vi "Display Console.vi"(8 "error in (no error)":errorcluster) -> (0 "error out":errorcluster)   [LabVIEW 2017]
uses:
  Type Definitions/Display Data.ctl
  Type Definitions/DB Record.ctl
  Type Definitions/Display Console States.ctl
  Type Definitions/Queue FG Options.ctl
panel:
  out "Card Read":bool
  out "Message Screen":string
  out "Current Transaction":string
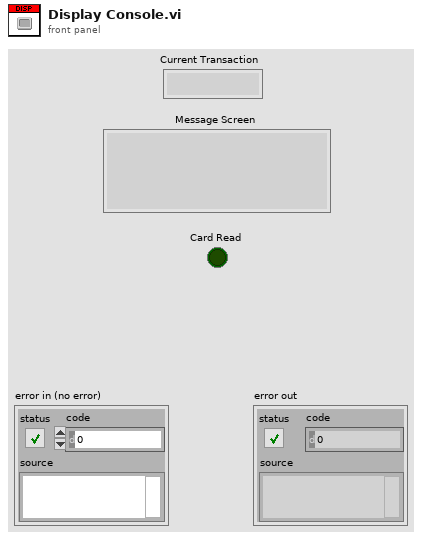
[diagram p1: front panel]
types:
  T1 = typedef "Display Data.ctl" = cluster{"Message Text":string, "DB Record":T2, "Card Read":bool, "Display Console States":T3}
  T2 = typedef "DB Record.ctl" = cluster{"Account":i32, "First Name":string, "Last Name":string, "Balance":fxp<+/-,64,35>}
  T3 = typedef "Display Console States.ctl" = enum16{"Timeout", "Initial", "Login", "Invalid Login", "Idle", "Balance Inquiry", "Deposit", "Withdrawal", "Fast Cash", "Withdrawal Failed", "Withdrawal Complete", "Terminate", "Shutdown"}
  T4 = typedef "Queue FG Options.ctl" = enum16{"Set", "Get", "Read", "Write", "Destroy"}
  T5 = typedef "Display Console Message.ctl" = cluster{"Message Info":T3, "Message Data":variant}
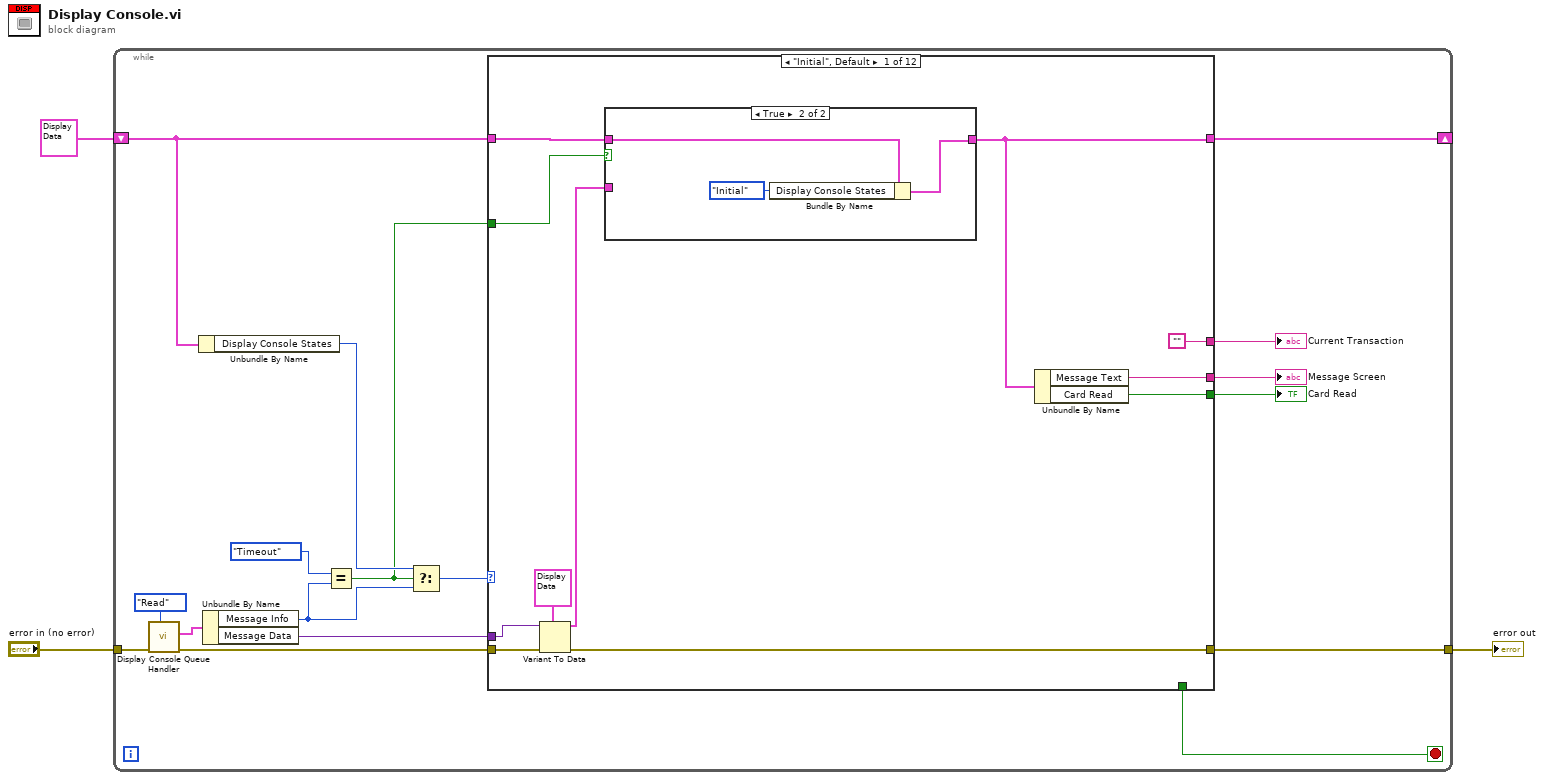
[diagram p0: block diagram]
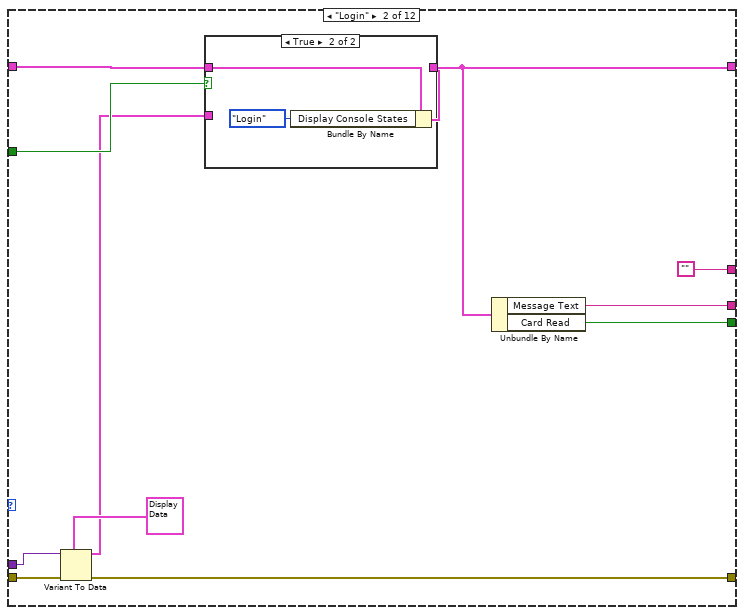
[diagram p3: hidden frame]
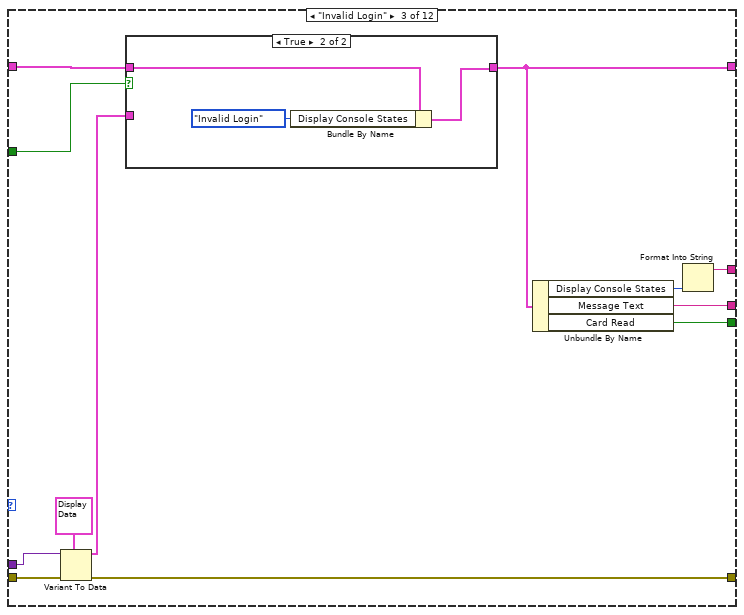
[diagram p5: hidden frame]
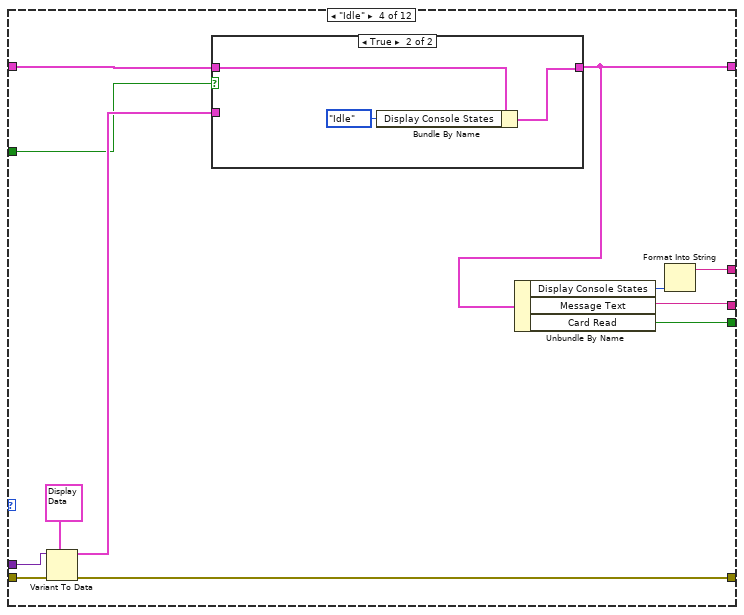
[diagram p7: hidden frame]
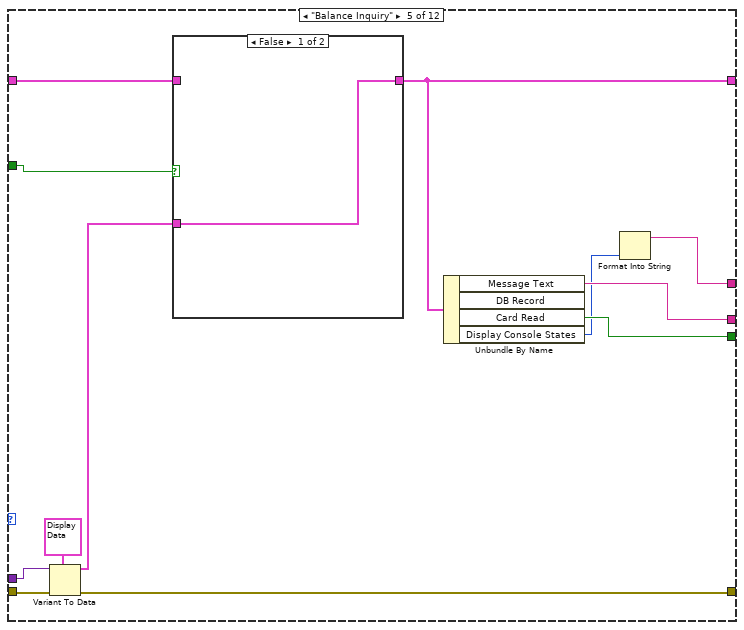
[diagram p9: hidden frame]
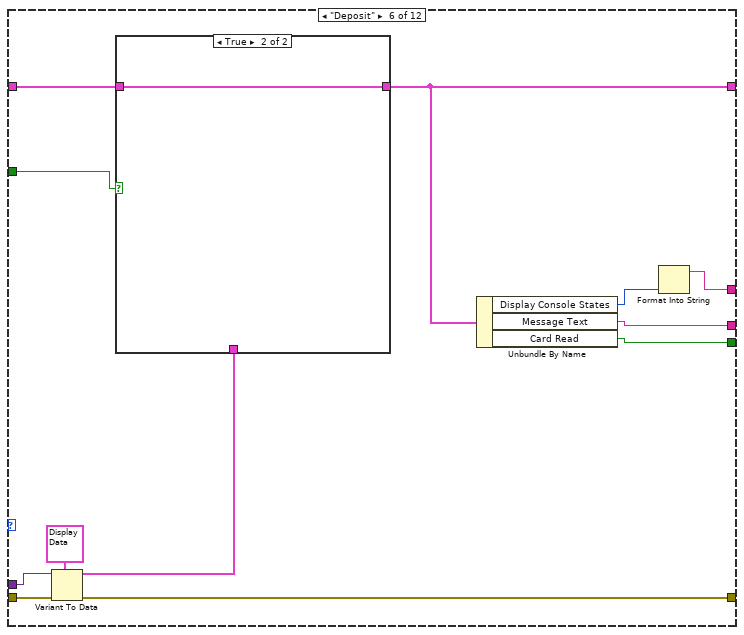
[diagram p11: hidden frame]
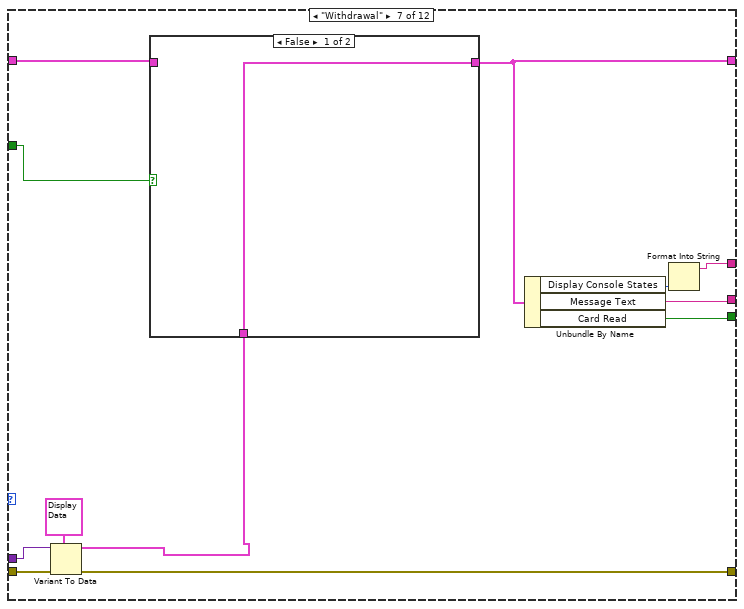
[diagram p13: hidden frame]
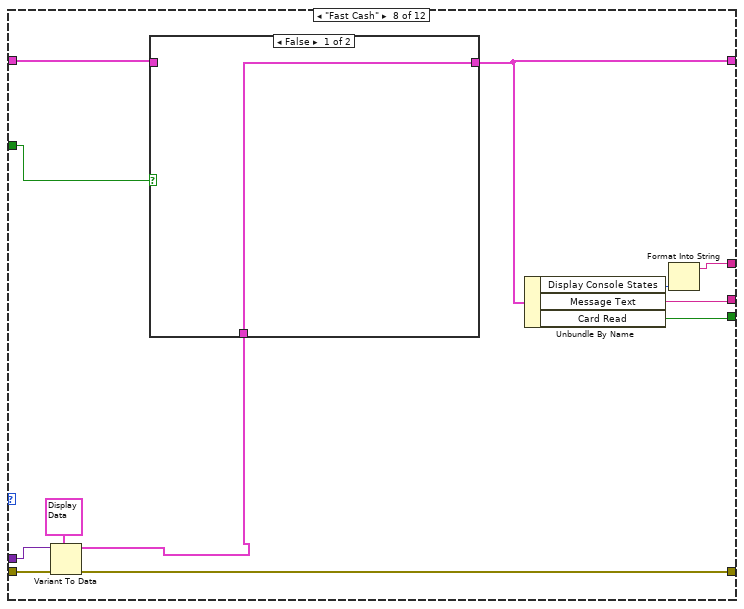
[diagram p15: hidden frame]
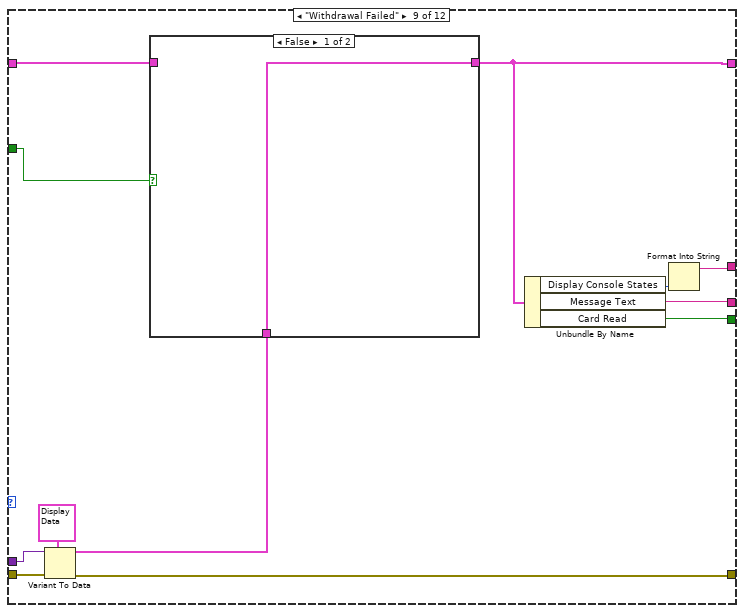
[diagram p17: hidden frame]
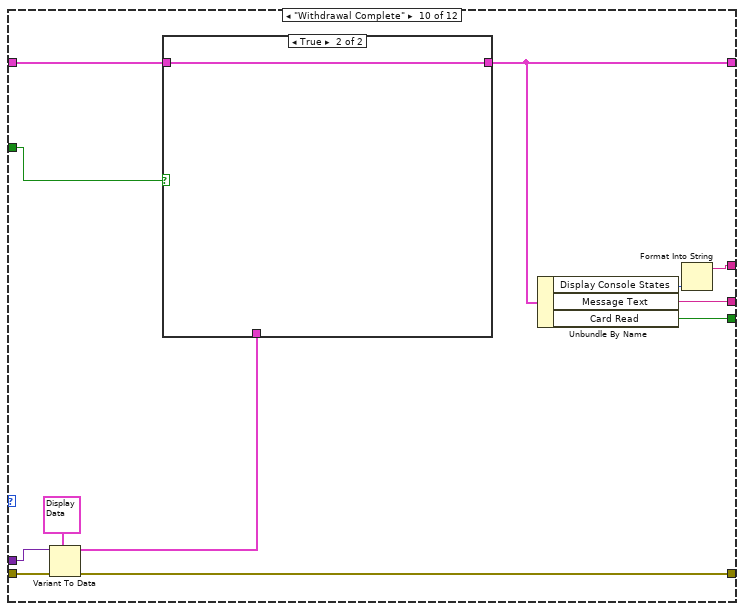
[diagram p19: hidden frame]
diagram:
  n1 = while {
    tunnel: "error in (no error)" -> [w19]
    tunnel: [w15] -> w2
    shift-right: [w10] -> _
    shift-left: T1 {"Message Text"="", "DB Record"={"Account"=0, "First Name"="", "Last Name"="", "Balance"=0.0}, "Card Read"=FALSE, "Display Console States"=enum."Timeout"} ("Display Data") -> [w5]
    stop <- w14 stop-if-true
    n2 = call "Display Console Queue Handler.vi"("Action"=Queue_FG_Options."Read", "error in (no error)"=w19) -> ("error out"=w16:errorcluster, "Message out"=w18:T5)  [unwired: 7 in, 1 out]
    n3 = Unbundle By Name(w5) -> ("Display Console States"=w6:T3)
    n4 = Unbundle By Name(w18) -> ("Message Info"=w8:T3, "Message Data"=w17:variant)
    n5 = Equal?(x=Display_Console_States."Timeout" ("Display Console States"), y=w8) -> (x = y?=w4:bool)
    n6 = Select(t=w6, s=w4, f=w8) -> (s? t:f=w7:T3)
    n7 = case shown="\"Initial\", Default" w7 {
      selector: w7 -> [_ _ _ _ _ _ _ _ _ _ _ w186]
      tunnel: w17 -> [w31 w46 w62 w75 w91 w105 w119 w133 w147 w161 w175 w185]
      tunnel: w16 -> [w30 w45 w61 w77 w93 w107 w121 w135 w149 w163 w177 w188]
      tunnel: [w29 w44 w60 w76 w92 w106 w120 w134 w148 w162 w176 w187] -> w15
      tunnel: [_ _ _ _ _ _ _ _ _ _ _ TRUE] -> w14
      tunnel: [w26 w41 w57 w69 w85 w100 w113 w127 w141 w154 w168 w183] -> w13
      tunnel: ["" "" w51 w70 w83 w97 w114 w128 w142 w155 w169 w182] -> w12
      tunnel: [w27 w42 w58 w68 w86 w99 w112 w126 w140 w153 w167 w184] -> w11
      tunnel: w5 -> [w24 w39 w55 w74 w90 w104 w116 w130 w145 w160 w174 w181]
      tunnel: [w22 w37 w53 w71 w87 w101 w115 w129 w143 w157 w171 w181] -> w10
      tunnel: w4 -> [w25 w40 w56 w67 w89 w102 w111 w125 w144 w158 w172 _]
      frame "Initial", Default {
        n8 = Variant To Data(error in=w30, type=T1 {"Message Text"="", "DB Record"={"Account"=0, "First Name"="", "Last Name"="", "Balance"=0.0}, "Card Read"=FALSE, "Display Console States"=enum."Timeout"} ("Display Data"), Variant=w31) -> (data=w23:T1, error out=w29:errorcluster)
        n9 = case shown="True" w25 {
          tunnel: w24 -> [_ w35]
          tunnel: [w32 w33] -> w22
          tunnel: w23 -> [w32 _]
          frame False {
          }
          frame True {
            n10 = Bundle By Name(cluster=w35, "Display Console States"=Display_Console_States."Initial") -> (w33:T1)
          }
        }
        n11 = Unbundle By Name(w22) -> ("Message Text"=w26:string, "Card Read"=w27:bool)
      }
      frame "Login" {
        n12 = Variant To Data(error in=w45, type=T1 {"Message Text"="", "DB Record"={"Account"=0, "First Name"="", "Last Name"="", "Balance"=0.0}, "Card Read"=FALSE, "Display Console States"=enum."Timeout"} ("Display Data"), Variant=w46) -> (data=w38:T1, error out=w44:errorcluster)
        n13 = case shown="True" w40 {
          tunnel: w39 -> [_ w50]
          tunnel: [w47 w48] -> w37
          tunnel: w38 -> [w47 _]
          frame False {
          }
          frame True {
            n14 = Bundle By Name(cluster=w50, "Display Console States"=Display_Console_States."Login") -> (w48:T1)
          }
        }
        n15 = Unbundle By Name(w37) -> ("Message Text"=w41:string, "Card Read"=w42:bool)
      }
      frame "Invalid Login" {
        n16 = Variant To Data(error in=w61, type=T1 {"Message Text"="", "DB Record"={"Account"=0, "First Name"="", "Last Name"="", "Balance"=0.0}, "Card Read"=FALSE, "Display Console States"=enum."Timeout"} ("Display Data"), Variant=w62) -> (data=w54:T1, error out=w60:errorcluster)
        n17 = case shown="True" w56 {
          tunnel: w55 -> [_ w66]
          tunnel: [w63 w64] -> w53
          tunnel: w54 -> [w63 _]
          frame False {
          }
          frame True {
            n18 = Bundle By Name(cluster=w66, "Display Console States"=Display_Console_States."Invalid Login") -> (w64:T1)
          }
        }
        n19 = Unbundle By Name(w53) -> ("Display Console States"=w52:T3, "Message Text"=w57:string, "Card Read"=w58:bool)
        n20 = Format Into String(w52) -> (resulting string=w51:string)  [unwired: 3 in, 1 out]
      }
      frame "Idle" {
        n21 = Variant To Data(error in=w77, type=T1 {"Message Text"="", "DB Record"={"Account"=0, "First Name"="", "Last Name"="", "Balance"=0.0}, "Card Read"=FALSE, "Display Console States"=enum."Timeout"} ("Display Data"), Variant=w75) -> (data=w73:T1, error out=w76:errorcluster)
        n22 = case shown="True" w67 {
          tunnel: w74 -> [_ w82]
          tunnel: [w79 w80] -> w71
          tunnel: w73 -> [w79 _]
          frame False {
          }
          frame True {
            n23 = Bundle By Name(cluster=w82, "Display Console States"=Display_Console_States."Idle") -> (w80:T1)
          }
        }
        n24 = Unbundle By Name(w71) -> ("Display Console States"=w72:T3, "Message Text"=w69:string, "Card Read"=w68:bool)
        n25 = Format Into String(w72) -> (resulting string=w70:string)  [unwired: 3 in, 1 out]
      }
      frame "Balance Inquiry" {
        n26 = Variant To Data(error in=w93, type=T1 {"Message Text"="", "DB Record"={"Account"=0, "First Name"="", "Last Name"="", "Balance"=0.0}, "Card Read"=FALSE, "Display Console States"=enum."Timeout"} ("Display Data"), Variant=w91) -> (data=w88:T1, error out=w92:errorcluster)
        n27 = case shown="False" w89 {
          tunnel: [w95 w96] -> w87
          tunnel: w90 -> [_ w96]
          tunnel: w88 -> [w95 _]
          frame False {
          }
          frame True {
          }
        }
        n28 = Unbundle By Name(w87) -> ("Message Text"=w85:string, "Card Read"=w86:bool, "Display Console States"=w84:T3)  [unwired: 1 out]
        n29 = Format Into String(w84) -> (resulting string=w83:string)  [unwired: 3 in, 1 out]
      }
      frame "Deposit" {
        n30 = Variant To Data(error in=w107, type=T1 {"Message Text"="", "DB Record"={"Account"=0, "First Name"="", "Last Name"="", "Balance"=0.0}, "Card Read"=FALSE, "Display Console States"=enum."Timeout"} ("Display Data"), Variant=w105) -> (data=w103:T1, error out=w106:errorcluster)
        n31 = case shown="True" w102 {
          tunnel: [w109 w110] -> w101
          tunnel: w104 -> [_ w110]
          tunnel: w103 -> [w109 _]
          frame False {
          }
          frame True {
          }
        }
        n32 = Unbundle By Name(w101) -> ("Display Console States"=w98:T3, "Message Text"=w100:string, "Card Read"=w99:bool)
        n33 = Format Into String(w98) -> (resulting string=w97:string)  [unwired: 3 in, 1 out]
      }
      frame "Withdrawal" {
        n34 = Variant To Data(error in=w121, type=T1 {"Message Text"="", "DB Record"={"Account"=0, "First Name"="", "Last Name"="", "Balance"=0.0}, "Card Read"=FALSE, "Display Console States"=enum."Timeout"} ("Display Data"), Variant=w119) -> (data=w117:T1, error out=w120:errorcluster)
        n35 = case shown="False" w111 {
          tunnel: w116 -> [_ w124]
          tunnel: [w123 w124] -> w115
          tunnel: w117 -> [w123 _]
          frame False {
          }
          frame True {
          }
        }
        n36 = Unbundle By Name(w115) -> ("Display Console States"=w118:T3, "Message Text"=w113:string, "Card Read"=w112:bool)
        n37 = Format Into String(w118) -> (resulting string=w114:string)  [unwired: 3 in, 1 out]
      }
      frame "Fast Cash" {
        n38 = Variant To Data(error in=w135, type=T1 {"Message Text"="", "DB Record"={"Account"=0, "First Name"="", "Last Name"="", "Balance"=0.0}, "Card Read"=FALSE, "Display Console States"=enum."Timeout"} ("Display Data"), Variant=w133) -> (data=w131:T1, error out=w134:errorcluster)
        n39 = case shown="False" w125 {
          tunnel: w130 -> [_ w138]
          tunnel: [w137 w138] -> w129
          tunnel: w131 -> [w137 _]
          frame False {
          }
          frame True {
          }
        }
        n40 = Unbundle By Name(w129) -> ("Display Console States"=w132:T3, "Message Text"=w127:string, "Card Read"=w126:bool)
        n41 = Format Into String(w132) -> (resulting string=w128:string)  [unwired: 3 in, 1 out]
      }
      frame "Withdrawal Failed" {
        n42 = Variant To Data(error in=w149, type=T1 {"Message Text"="", "DB Record"={"Account"=0, "First Name"="", "Last Name"="", "Balance"=0.0}, "Card Read"=FALSE, "Display Console States"=enum."Timeout"} ("Display Data"), Variant=w147) -> (data=w139:T1, error out=w148:errorcluster)
        n43 = case shown="False" w144 {
          tunnel: w145 -> [_ w152]
          tunnel: [w151 w152] -> w143
          tunnel: w139 -> [w151 _]
          frame False {
          }
          frame True {
          }
        }
        n44 = Unbundle By Name(w143) -> ("Display Console States"=w146:T3, "Message Text"=w141:string, "Card Read"=w140:bool)
        n45 = Format Into String(w146) -> (resulting string=w142:string)  [unwired: 3 in, 1 out]
      }
      frame "Withdrawal Complete" {
        n46 = Variant To Data(error in=w163, type=T1 {"Message Text"="", "DB Record"={"Account"=0, "First Name"="", "Last Name"="", "Balance"=0.0}, "Card Read"=FALSE, "Display Console States"=enum."Timeout"} ("Display Data"), Variant=w161) -> (data=w159:T1, error out=w162:errorcluster)
        n47 = case shown="True" w158 {
          tunnel: w160 -> [_ w166]
          tunnel: [w165 w166] -> w157
          tunnel: w159 -> [w165 _]
          frame False {
          }
          frame True {
          }
        }
        n48 = Unbundle By Name(w157) -> ("Display Console States"=w156:T3, "Message Text"=w154:string, "Card Read"=w153:bool)
        n49 = Format Into String(w156) -> (resulting string=w155:string)  [unwired: 3 in, 1 out]
      }
      frame "Terminate" {
        n50 = Variant To Data(error in=w177, type=T1 {"Message Text"="", "DB Record"={"Account"=0, "First Name"="", "Last Name"="", "Balance"=0.0}, "Card Read"=FALSE, "Display Console States"=enum."Timeout"} ("Display Data"), Variant=w175) -> (data=w173:T1, error out=w176:errorcluster)
        n51 = case shown="False" w172 {
          tunnel: w174 -> [_ w180]
          tunnel: [w179 w180] -> w171
          tunnel: w173 -> [w179 _]
          frame False {
          }
          frame True {
          }
        }
        n52 = Unbundle By Name(w171) -> ("Display Console States"=w170:T3, "Message Text"=w168:string, "Card Read"=w167:bool)
        n53 = Format Into String(w170) -> (resulting string=w169:string)  [unwired: 3 in, 1 out]
      }
      frame "Shutdown" {
        n54 = Format Into String(w186) -> (resulting string=w182:string)  [unwired: 3 in, 1 out]
        n55 = Variant To Data(error in=w188, type=T1 {"Message Text"="", "DB Record"={"Account"=0, "First Name"="", "Last Name"="", "Balance"=0.0}, "Card Read"=FALSE, "Display Console States"=enum."Timeout"} ("Display Data"), Variant=w185) -> (data=w189:T1, error out=w187:errorcluster)
        n56 = Unbundle By Name(w189) -> ("Message Text"=w183:string, "Card Read"=w184:bool)  [unwired: 1 out]
      }
    }
    "Current Transaction" <- w12
    "Message Screen" <- w13
    "Card Read" <- w11
  }
  "error out" <- w2
